vi "SSL Geometry Data.vi"(5 "Version":string(combo)="Auto", 7 "Optional":bool, 8 "error in":errorcluster, 9 "Array":u8[](array[numeric]) format="%02x") -> (0 "error out":errorcluster, 2 "Geometry Camera Calibration":T1, 3 "Field Size":refnum<class "Field.lvclass">)   [LabVIEW 2018]
uses:
  Controls/SSL Geometry Camera Calibration.ctl
  Field_class/Field.lvclass
  Varint Decoder uint32.vi
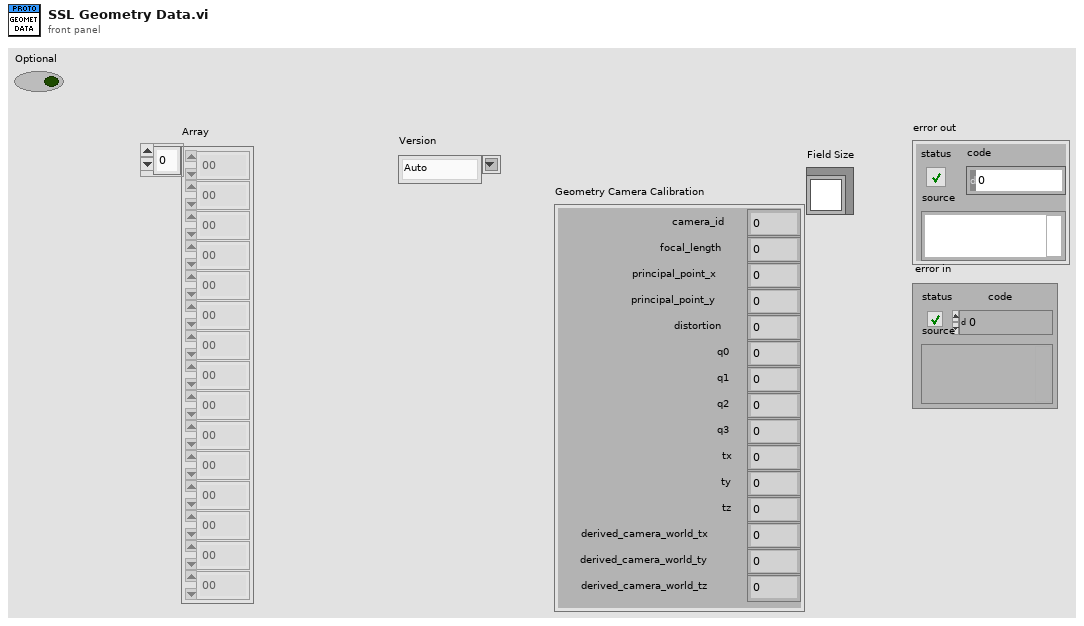
[diagram p1: front panel]
types:
  T1 = typedef "SSL Geometry Camera Calibration.ctl" = cluster{"camera_id":u32, "focal_length":sgl, "principal_point_x":sgl, "principal_point_y":sgl, "distortion":sgl, "q0":sgl, "q1":sgl, "q2":sgl, "q3":sgl, "tx":sgl, "ty":sgl, "tz":sgl, "derived_camera_world_tx":sgl, "derived_camera_world_ty":sgl, "derived_camera_world_tz":sgl}
  T2 = cluster{"[0]":sgl, "[1]":sgl, "[2]":sgl, "[3]":sgl, "[4]":sgl, "[5]":sgl, "[6]":sgl, "[7]":sgl, "[8]":sgl, "[9]":sgl, "[10]":sgl, "[11]":sgl, "[12]":sgl, "[13]":sgl, "[14]":sgl}
  T3 = cluster{"[0]":u32, "[1]":u32, "[2]":u32, "[3]":u32, "[4]":u32, "[5]":u32, "[6]":u32, "[7]":u32, "[8]":u32, "[9]":u32, "[10]":u32, "[11]":u32, "[12]":u32, "[13]":u32}
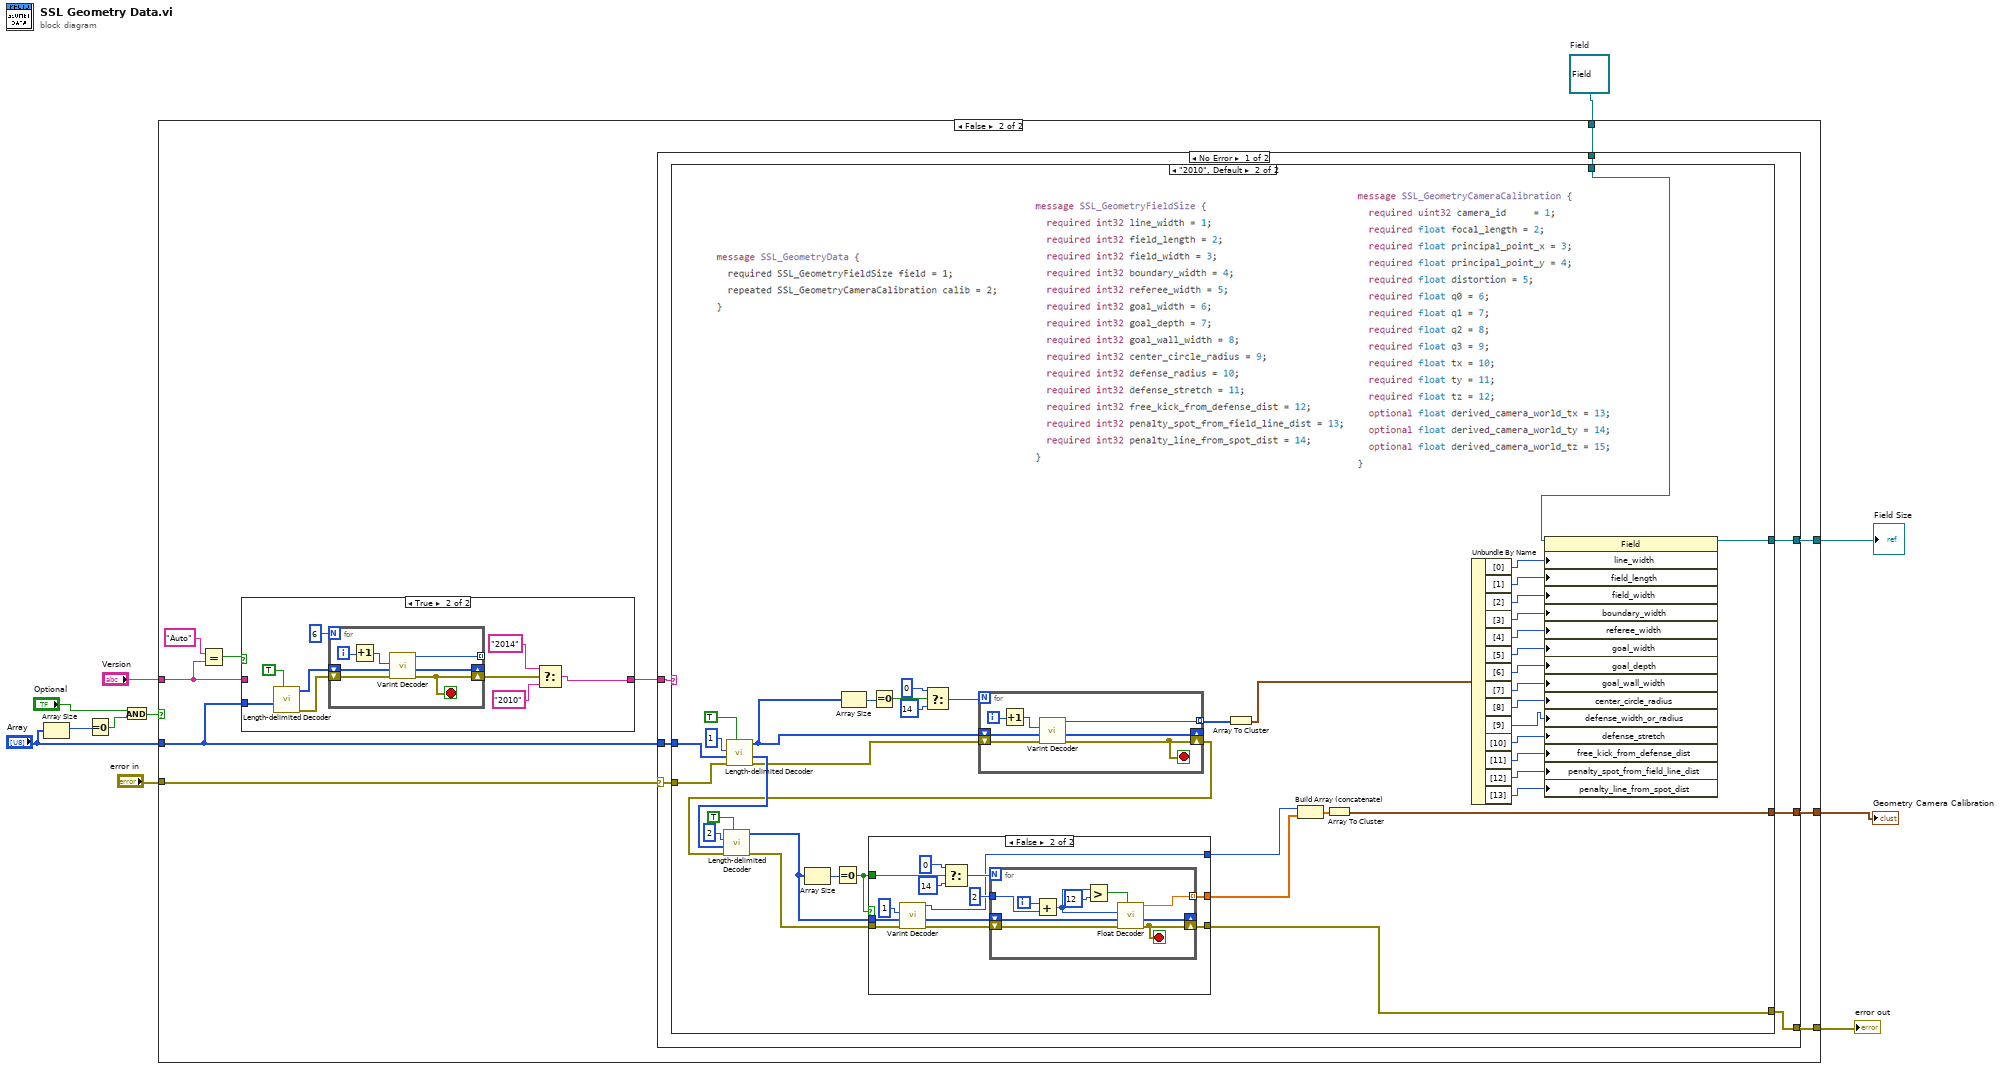
[diagram p0: block diagram]
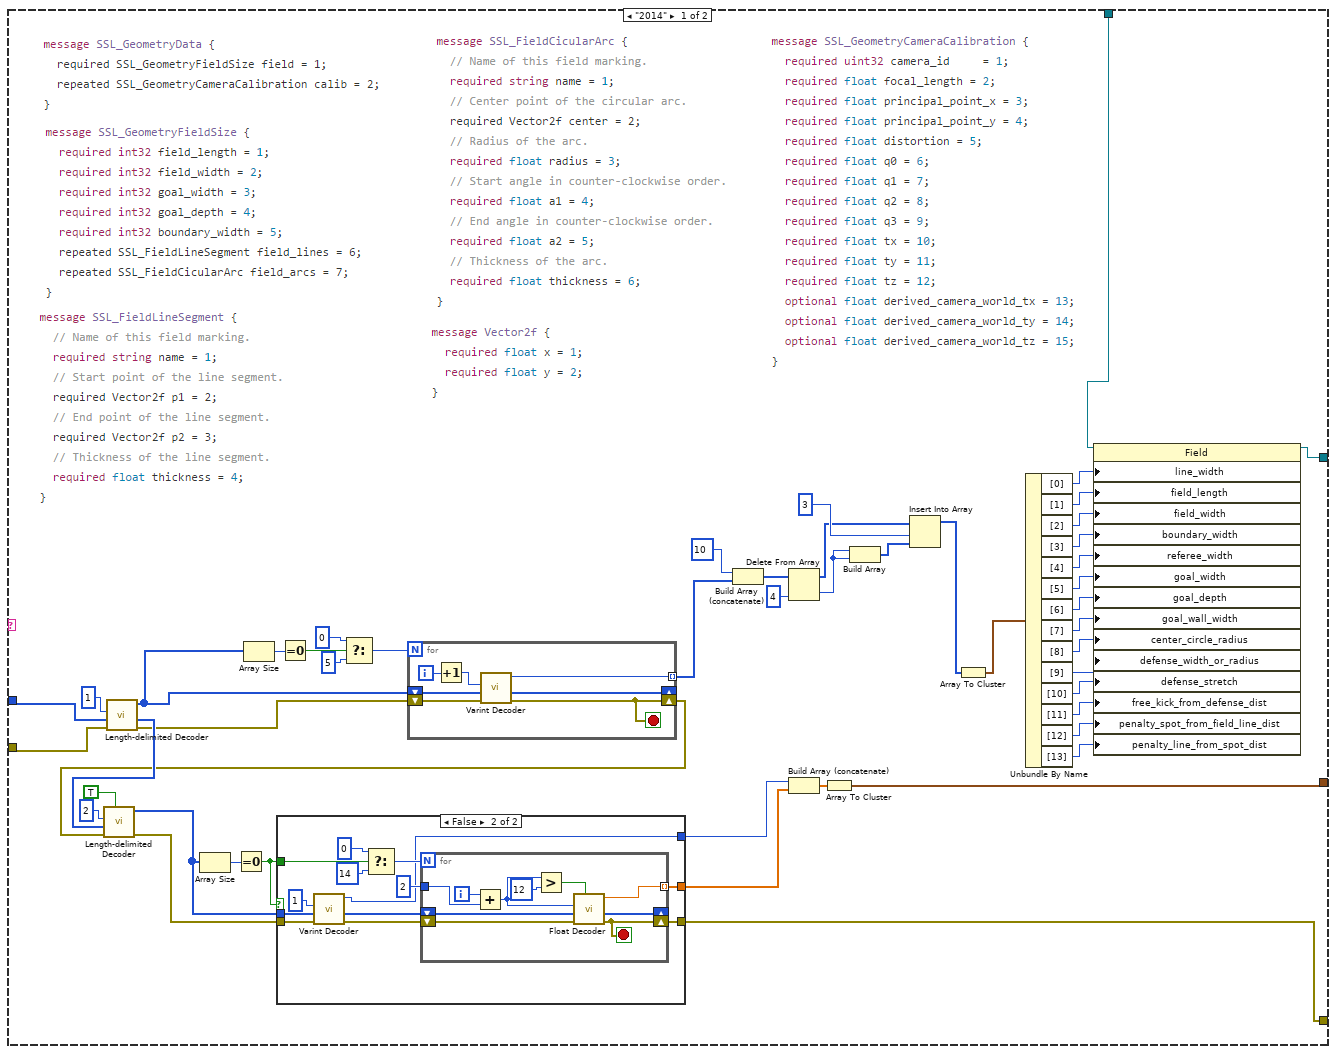
[diagram p4: hidden frame]
diagram:
  w1 = refnum<class "Field.lvclass"> refnum  # Field
  n1 = Array Size(array="Array") -> (size(s)=w5:i32)
  n2 = Equal To 0?(x=w5) -> (x = 0?=w6:bool)
  n3 = And(x="Optional", y=w6) -> (x .and. y?=w7:bool)
  n4 = case shown="False" w7 {
    tunnel: "error in" -> [w13 w23]
    tunnel: [w13 w22] -> w10
    tunnel: "Array" -> [_ w16]
    tunnel: "Version" -> [_ w18]
    tunnel: [_ w21] -> w3
    tunnel: [w12 w15] -> w2
    tunnel: w1 -> [w12 w14]
    frame True {
    }
    frame False {
      n5 = Equal?(x="Auto", y=w18) -> (x = y?=w19:bool)
      n6 = case shown="True" w19 {
        tunnel: w18 -> [w24 _]
        tunnel: [w24 w27] -> w17
        tunnel: w16 -> [_ w33]
        frame False {
        }
        frame True {
          n7 = call "Length-delimited Decoder.vi"("Optional"=TRUE, "Array"=w33) -> ("error out"=w31:errorcluster, "Length-delimited"=w32:u8[])  [unwired: 6 in, 2 out]
          n8 = for {
            N: 6 -> [_]
            tunnel: [w40] -> _ mode=indexing
            shift-right: [w39] -> _
            shift-left: w32 -> [w35]
            shift-right: [w37] -> w28
            shift-left: w31 -> [w38]
            i -> [w36]
            stop <- w37 stop-if-true
            n9 = Increment(x=w36) -> (x+1=w34:i32)
            n10 = call-poly "Varint Decoder.vi"("error in (no error)"=w38, "Array"=w35, "Key"=w34) -> ("error out"=w37:errorcluster, "array w/ subset deleted"=w39:u8[], "Varint"=w40:u32)  [unwired: 5 in, 1 out]
          }
          n11 = Select(t="2014" ("x"), s=w28, f="2010" ("x")) -> (s? t:f=w27:string)
        }
      }
      n12 = case shown="No Error" w23 {
        selector: w23 -> [w47 w201]
        tunnel: [w46 w201] -> w22
        tunnel: w16 -> [w45 _]
        tunnel: w17 -> [w44 _]
        tunnel: [w43 _] -> w21
        tunnel: [w42 _] -> w15
        tunnel: w14 -> [w41 _]
        frame No Error {
          n13 = case shown="\"2010\", Default" w44 {
            tunnel: w47 -> [w76 w169]
            tunnel: [w75 w158] -> w46
            tunnel: w45 -> [w77 w151]
            tunnel: [w74 w145] -> w43
            tunnel: [w49 w129] -> w42
            tunnel: w41 -> [w48 w128]
            frame "2014" {
              n14 = call "Length-delimited Decoder.vi"("error in (no error)"=w76, "Array"=w77, "Key"=1) -> ("error out"=w85:errorcluster, "array w/ subset deleted"=w87:u8[], "Length-delimited"=w94:u8[])  [unwired: 5 in, 1 out]
              n15 = Array Size(array=w94) -> (size(s)=w93:i32)
              n16 = Equal To 0?(x=w93) -> (x = 0?=w92:bool)
              n17 = Select(t=0, s=w92, f=5) -> (s? t:f=w89:i32)
              n18 = for {
                N: w89 -> [_]
                tunnel: [w127] -> w72 mode=indexing
                shift-right: [w126] -> _
                shift-left: w94 -> [w122]
                shift-right: [w124] -> w84
                shift-left: w85 -> [w125]
                i -> [w123]
                stop <- w124 stop-if-true
                n19 = Increment(x=w123) -> (x+1=w121:i32)
                n20 = call-poly "Varint Decoder.vi"("error in (no error)"=w125, "Array"=w122, "Key"=w121) -> ("error out"=w124:errorcluster, "array w/ subset deleted"=w126:u8[], "Varint"=w127:u32)  [unwired: 5 in, 1 out]
              }
              n21 = call "Length-delimited Decoder.vi"("Optional"=TRUE, "error in (no error)"=w84, "Array"=w87, "Key"=2) -> ("error out"=w83:errorcluster, "Length-delimited"=w78:u8[])  [unwired: 4 in, 2 out]
              n22 = Array Size(array=w78) -> (size(s)=w88:i32)
              n23 = Equal To 0?(x=w88) -> (x = 0?=w82:bool)
              n24 = case shown="False" w82 {
                tunnel: w82 -> [_ w110]
                tunnel: [w97 w106] -> w75
                tunnel: [_ w103] -> w80
                tunnel: w83 -> [w97 w101]
                tunnel: w78 -> [_ w100]
                tunnel: [_ w98] -> w81
                frame True {
                }
                frame False {
                  n25 = call-poly "Varint Decoder.vi"("error in (no error)"=w101, "Array"=w100, "Key"=1) -> ("error out"=w102:errorcluster, "array w/ subset deleted"=w105:u8[], "Varint"=w98:u32)  [unwired: 5 in, 1 out]
                  n26 = Select(t=0, s=w110, f=14) -> (s? t:f=w107:i32)
                  n27 = for {
                    N: w107 -> [_]
                    tunnel: [w113] -> w103 mode=indexing
                    shift-right: [w120] -> _
                    shift-left: w105 -> [w112]
                    shift-right: [w118] -> w106
                    shift-left: w102 -> [w119]
                    tunnel: 2 ("y") -> [w114]
                    i -> [w116]
                    stop <- w118 stop-if-true
                    n28 = Add(x=w116, y=w114) -> (x+y=w115:i32)
                    n29 = Greater?(x=w115, y=12) -> (0:w111:bool)
                    n30 = call "Float Decoder.vi"("Optional"=w111, "error in (no error)"=w119, "Array"=w112, "Key"=w115) -> ("error out"=w118:errorcluster, "array w/ subset deleted"=w120:u8[], "Float"=w113:sgl)  [unwired: 4 in, 1 out]
                  }
                }
              }
              n31 = Build Array (concatenate)(u32 10 ("element"), w72) -> (w71:u32[])
              n32 = Delete From Array(array=w71, index=4) -> (deleted portion=w69:u32, array with subset deleted=w67:u32[])  [unwired: 1 in]
              n33 = Build Array (concatenate)(w81, w80) -> (w79:sgl[])
              n34 = Array To Cluster(array=w79) -> (cluster=w74:T2)
              n35 = Build Array(w69, w69) -> (w68:u32[])
              n36 = Insert Into Array(array=w67, index=3, new element=w68) -> (w65:u32[])
              n37 = Array To Cluster(array=w65) -> (cluster=w64:T3)
              n38 = Unbundle By Name(w64) -> ("[0]"=w63:u32, "[1]"=w62:u32, "[2]"=w61:u32, "[3]"=w60:u32, "[4]"=w59:u32, "[5]"=w58:u32, "[6]"=w57:u32, "[7]"=w56:u32, "[8]"=w55:u32, "[9]"=w54:u32, "[10]"=w53:u32, "[11]"=w52:u32, "[12]"=w51:u32, "[13]"=w50:u32)
              n39 = property class="Field"(reference=w48, "line_width"=w63, "field_length"=w62, "field_width"=w61, "boundary_width"=w60, "referee_width"=w59, "goal_width"=w58, "goal_depth"=w57, "goal_wall_width"=w56, "center_circle_radius"=w55, "defense_width_or_radius"=w54, "defense_stretch"=w53, "free_kick_from_defense_dist"=w52, "penalty_spot_from_field_line_dist"=w51, "penalty_line_from_spot_dist"=w50) -> (reference out=w49:refnum<class "Field.lvclass">)  [unwired: 1 in, 1 out]
            }
            frame "2010", Default {
              n40 = call "Length-delimited Decoder.vi"("Optional"=TRUE, "error in (no error)"=w169, "Array"=w151, "Key"=1) -> ("error out"=w155:errorcluster, "array w/ subset deleted"=w157:u8[], "Length-delimited"=w166:u8[])  [unwired: 4 in, 1 out]
              n41 = Array Size(array=w166) -> (size(s)=w165:i32)
              n42 = Equal To 0?(x=w165) -> (x = 0?=w164:bool)
              n43 = Select(t=0, s=w164, f=14) -> (s? t:f=w161:i32)
              n44 = for {
                N: w161 -> [_]
                tunnel: [w200] -> w160 mode=indexing
                shift-right: [w199] -> _
                shift-left: w166 -> [w195]
                shift-right: [w197] -> w154
                shift-left: w155 -> [w198]
                i -> [w196]
                stop <- w197 stop-if-true
                n45 = Increment(x=w196) -> (x+1=w194:i32)
                n46 = call-poly "Varint Decoder.vi"("error in (no error)"=w198, "Array"=w195, "Key"=w194) -> ("error out"=w197:errorcluster, "array w/ subset deleted"=w199:u8[], "Varint"=w200:u32)  [unwired: 5 in, 1 out]
              }
              n47 = call "Length-delimited Decoder.vi"("Optional"=TRUE, "error in (no error)"=w154, "Array"=w157, "Key"=2) -> ("error out"=w152:errorcluster, "Length-delimited"=w146:u8[])  [unwired: 4 in, 2 out]
              n48 = Array Size(array=w146) -> (size(s)=w159:i32)
              n49 = Equal To 0?(x=w159) -> (x = 0?=w150:bool)
              n50 = case shown="False" w150 {
                tunnel: w150 -> [_ w183]
                tunnel: [w170 w179] -> w158
                tunnel: [_ w176] -> w148
                tunnel: w152 -> [w170 w174]
                tunnel: w146 -> [_ w173]
                tunnel: [_ w171] -> w149
                frame True {
                }
                frame False {
                  n51 = call-poly "Varint Decoder.vi"("error in (no error)"=w174, "Array"=w173, "Key"=1) -> ("error out"=w175:errorcluster, "array w/ subset deleted"=w178:u8[], "Varint"=w171:u32)  [unwired: 5 in, 1 out]
                  n52 = Select(t=0, s=w183, f=14) -> (s? t:f=w180:i32)
                  n53 = for {
                    N: w180 -> [_]
                    tunnel: [w186] -> w176 mode=indexing
                    shift-right: [w193] -> _
                    shift-left: w178 -> [w185]
                    shift-right: [w191] -> w179
                    shift-left: w175 -> [w192]
                    tunnel: 2 ("y") -> [w187]
                    i -> [w189]
                    stop <- w191 stop-if-true
                    n54 = Add(x=w189, y=w187) -> (x+y=w188:i32)
                    n55 = Greater?(x=w188, y=12) -> (0:w184:bool)
                    n56 = call "Float Decoder.vi"("Optional"=w184, "error in (no error)"=w192, "Array"=w185, "Key"=w188) -> ("error out"=w191:errorcluster, "array w/ subset deleted"=w193:u8[], "Float"=w186:sgl)  [unwired: 4 in, 1 out]
                  }
                }
              }
              n57 = Array To Cluster(array=w160) -> (cluster=w130:T3)
              n58 = Build Array (concatenate)(w149, w148) -> (w147:sgl[])
              n59 = Array To Cluster(array=w147) -> (cluster=w145:T2)
              n60 = Unbundle By Name(w130) -> ("[0]"=w144:u32, "[1]"=w143:u32, "[2]"=w142:u32, "[3]"=w141:u32, "[4]"=w140:u32, "[5]"=w139:u32, "[6]"=w138:u32, "[7]"=w137:u32, "[8]"=w136:u32, "[9]"=w135:u32, "[10]"=w134:u32, "[11]"=w133:u32, "[12]"=w132:u32, "[13]"=w131:u32)
              n61 = property class="Field"(reference=w128, "line_width"=w144, "field_length"=w143, "field_width"=w142, "boundary_width"=w141, "referee_width"=w140, "goal_width"=w139, "goal_depth"=w138, "goal_wall_width"=w137, "center_circle_radius"=w136, "defense_width_or_radius"=w135, "defense_stretch"=w134, "free_kick_from_defense_dist"=w133, "penalty_spot_from_field_line_dist"=w132, "penalty_line_from_spot_dist"=w131) -> (reference out=w129:refnum<class "Field.lvclass">)  [unwired: 1 in, 1 out]
            }
          }
        }
        frame Error {
        }
      }
    }
  }
  "error out" <- w10
  "Geometry Camera Calibration" <- w3
  "Field Size" <- w2
